vi "CAT071_main_org.vi"() -> ()   [LabVIEW 2015]
uses:
  class.dbc/controls/dbc-signal.ctl
  class.dbc/controls/dbc-frame.ctl
  class.dbc/controls/dbc-cluster.ctl
  class.can.table/CAN_table.ctl
  class.dbc/controls/signals.result.ctl
  class.dbc/controls/signal.result.ctl
  subs/frame.type.ctl
  class.bFrameIO/bFrameIO.lvclass/bFrameIO.ctl
  class.dbc/dbc.lvclass/dbc.ctl
  class.bFrameIO/controls/input-states.ctl
  class.dbc/Read-active-frame-tag.vi
  class.dbc/Read-active-item-symbol.vi
  class.dbc/Read-active-item-tag.vi
  class.bFrameIO/wrt-fi-state.vi
  class.dbc/Write-active-item-tag.vi
  class.dbc/Write-active-item-symbol.vi
  class.dbc/Write-active-item-indent-lvl.vi
  class.dbc/Write-active-frame-tag.vi
  class.bFrameIO/read-baud-rate.vi
  class.bFrameIO/wrt-device.vi
  class.bFrameIO/Read-frameQ.vi
  class.bFrameIO/wrt-baud-rate.vi
  class.dbc/dbc.lvclass
  class.bFrameIO/bFrameIO.lvclass
  LEDarray/LEDarray.lvclass
  class.can.table/bAPPdata.lvclass
panel:
  in  "Interface":refnum<k21>
  in  "dbc.alias":string="CAT071"
  out "Path":path caption="Open .dbc file"
  in  "CAT.071":enum32{"DBC", "table"}(tab)
  in  "attributes":T1(tab)
  out "CAN.table":T2
  out "dbc.cluster":T3={"Name"="", "Baud Rate"=125000, "Application Protocol"=enum."None", "Comment"=""}
  out "signal.results":T4 {"payload" format="%3d"}
  out "dbc.frame":T6={"Comment"="", "Extended Identifier?"=FALSE, "Transmit Time"=0.0, "Timing Type"=1, "Payload Length"=8, "Identifier"=1, "Frame name"="frame1"} {"Timing Type" items=["Cyclic Data", "Event Data", "Cyclic Remote", "Event Remote"]; "Identifier" format="%010x"}
  out "payload":bool[][](array[boolean])
  in  "send.frame":bool
  in  "frame.type":T7
  in  "send.signal":bool
  out "leds":picture
  out "output.signal":T8={"Comment"="", "Byte Order"=0, "Data Type"=1, "Number of Bits"=8, "Start Bit"=0, "Unit"="V", "Default Value"=0.0, "Minimum Value"=0.0, "Maximum Value"=256.0, "Scaling Offset"=0.0, "Scaling Factor"=1.0, "Signal name"="signal1"} {"Byte Order" items=["Little Endian", "Big Endian"]; "Data Type" items=["Signed", "Unsigned", "IEEE Float"]}
  out "signal.payload":u32
  in  "hslide":dbl(slide) min=0.0 max=250.0 scale=0.0..250.0
  out "output.signal 2":T8={"Comment"="", "Byte Order"=0, "Data Type"=1, "Number of Bits"=8, "Start Bit"=0, "Unit"="V", "Default Value"=0.0, "Minimum Value"=0.0, "Maximum Value"=256.0, "Scaling Offset"=0.0, "Scaling Factor"=1.0, "Signal name"="signal1"} {"Byte Order" items=["Little Endian", "Big Endian"]; "Data Type" items=["Signed", "Unsigned", "IEEE Float"]}
  out "signal.payload 2":u32 caption="signal.payload"
  out "payload 2":bool[][](array[boolean]) caption="payload"
  in  "database":string(tree)
  # "CAT 071 \nMarquardt Inc @2017\nK.R. Bergerstock"
  # "CLUSTER"
  # "FRAME"
  # "SIGNAL"
  # "SIGNAL"
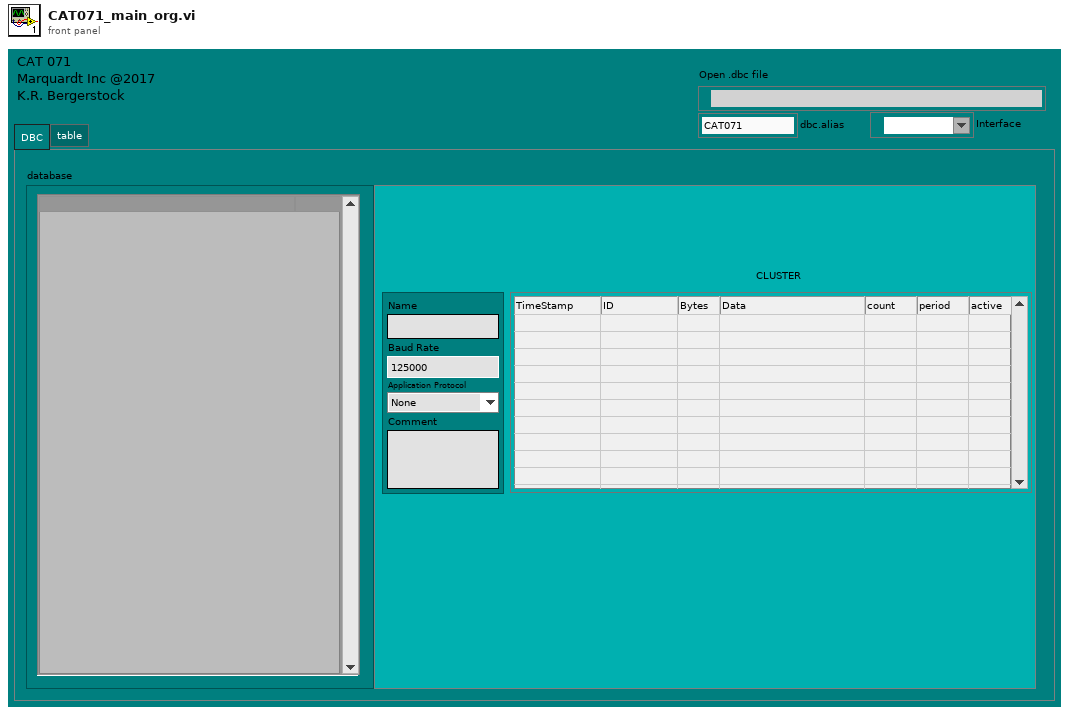
[diagram p1: front panel]
types:
  T1 = enum32{"cluster", "frame", "outp.signal", "inp.signal"}
  T2 = typedef "CAN_table.ctl" = string[][]
  T3 = typedef "dbc-cluster.ctl" = cluster{"Name":string, "Baud Rate":u32, "Application Protocol":enum16{"None", "J1939"}, "Comment":string}
  T4 = typedef "signals.result.ctl" = T5[]
  T5 = typedef "signal.result.ctl" = cluster{"Signal name":string, "payload":u8}
  T6 = typedef "dbc-frame.ctl" = cluster{"Comment":string, "Extended Identifier?":bool, "Transmit Time":dbl, "Timing Type":u32, "Payload Length":u32, "Identifier":u32, "Frame name":string}
  T7 = typedef "frame.type.ctl" = enum16{"FRAME NOT DEFINED", "DUT OUTPUT FRAME", "DUT INPUT FRAME"}
  T8 = typedef "dbc-signal.ctl" = cluster{"Comment":string, "Byte Order":u32, "Data Type":u32, "Number of Bits":u32, "Start Bit":u32, "Unit":string, "Default Value":dbl, "Minimum Value":dbl, "Maximum Value":dbl, "Scaling Offset":dbl, "Scaling Factor":dbl, "Signal name":string}
  T9 = typedef "bFrameIO.lvclass/input-states.ctl" = enum16{"idle", "start", "run", "stop", "exit"}
  T10 = typedef "frame-defination.ctl" = cluster{"CAN.frame":T6, "frame.type":T7}
  T11 = typedef "LVPoint32TypeDef.ctl" = cluster{"Horizontal":i32, "Vertical":i32}
  T12 = typedef "LVRectTypeDef.ctl" = cluster{"Left":i16, "Top":i16, "Right":i16, "Bottom":i16}
  T13 = typedef "XNET Frame CAN.ctl" = cluster{"timestamp":timestamp, "payload":u8[], "identifier":u32, "type":T14, "extended?":bool, "echo?":bool}
  T14 = typedef "XNET Frame Type CAN.ctl" = u8
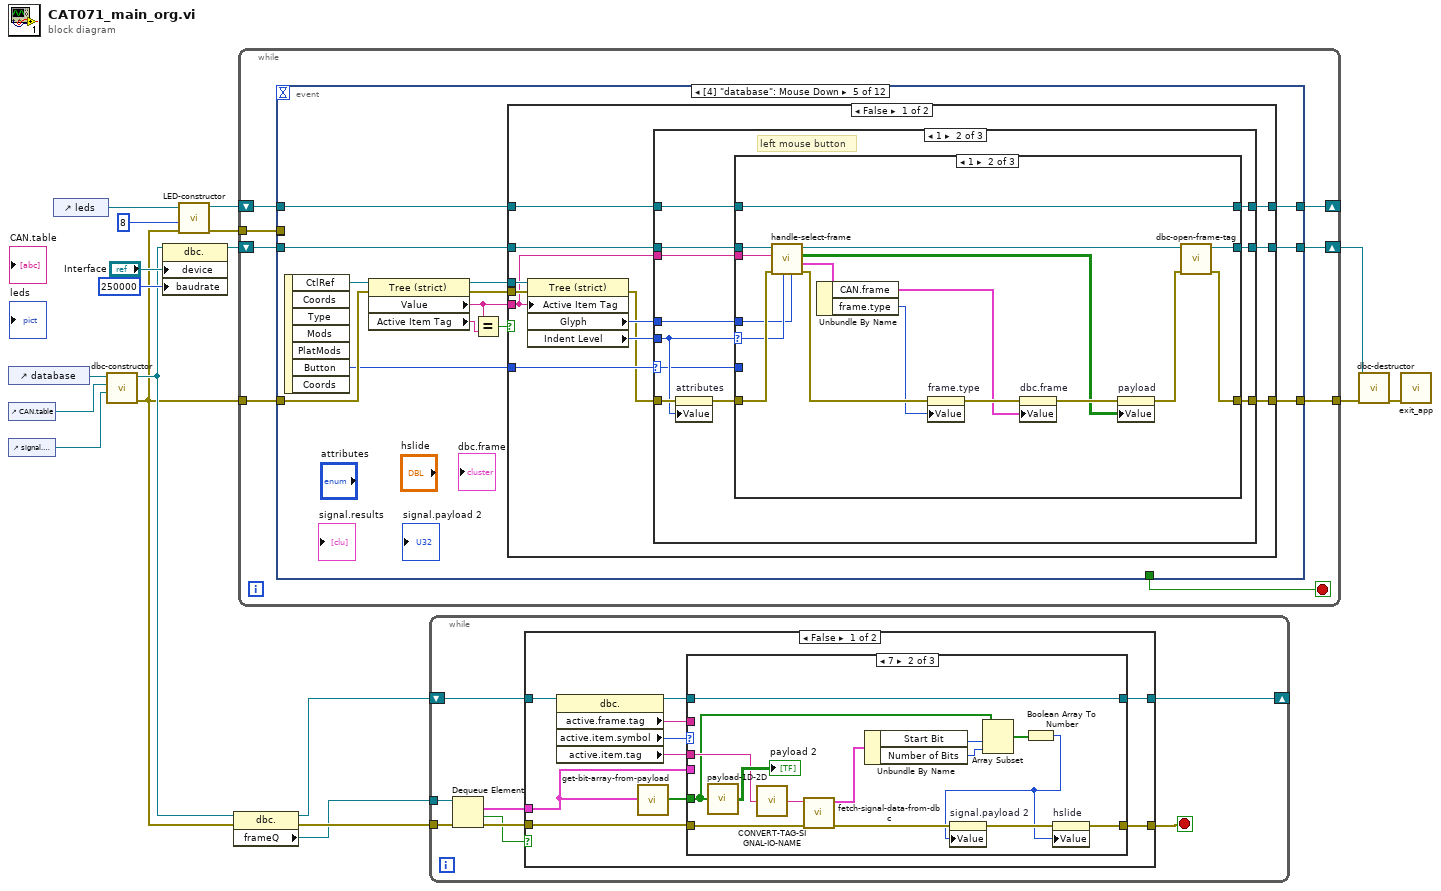
[diagram p0: block diagram]
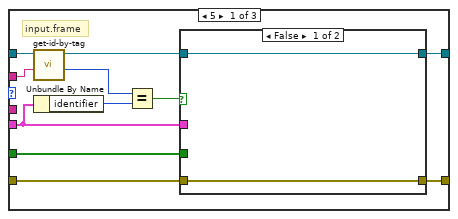
[diagram p2: hidden frame]
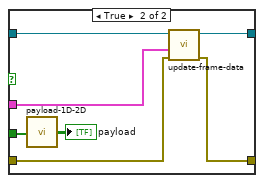
[diagram p3: hidden frame]
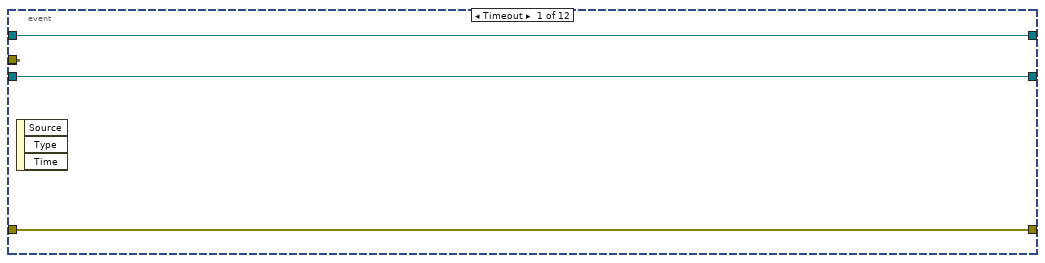
[diagram p6: hidden frame]
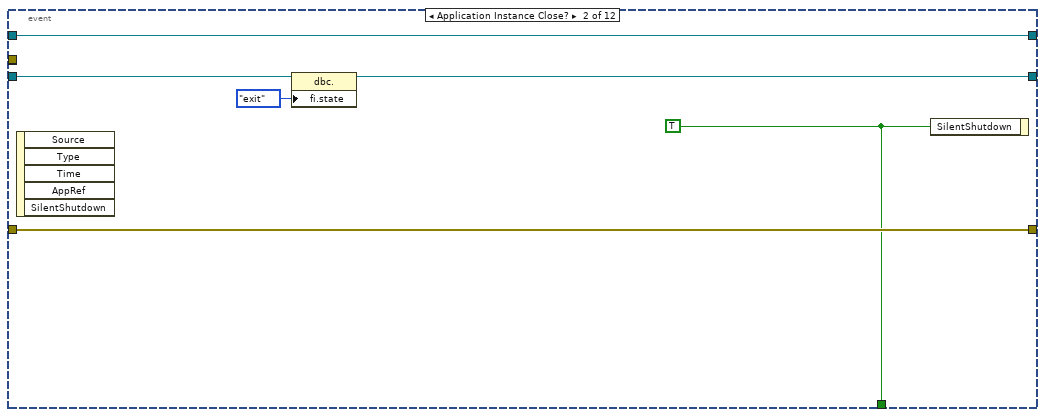
[diagram p7: hidden frame]
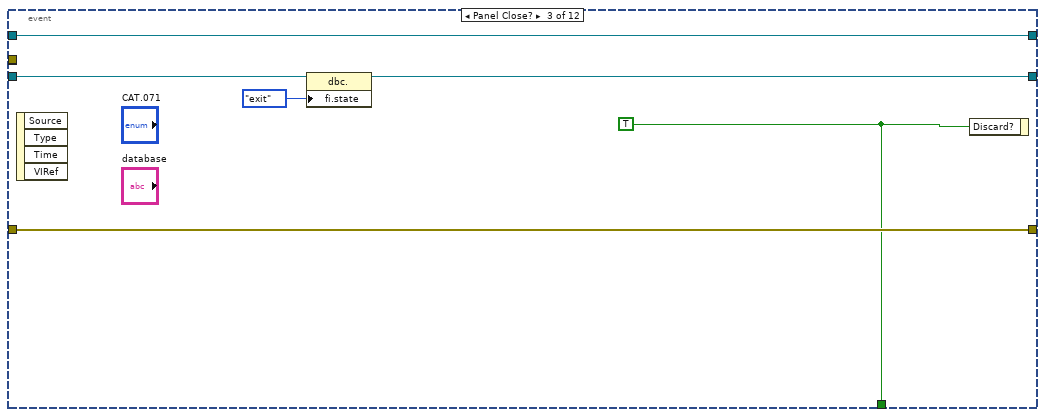
[diagram p8: hidden frame]
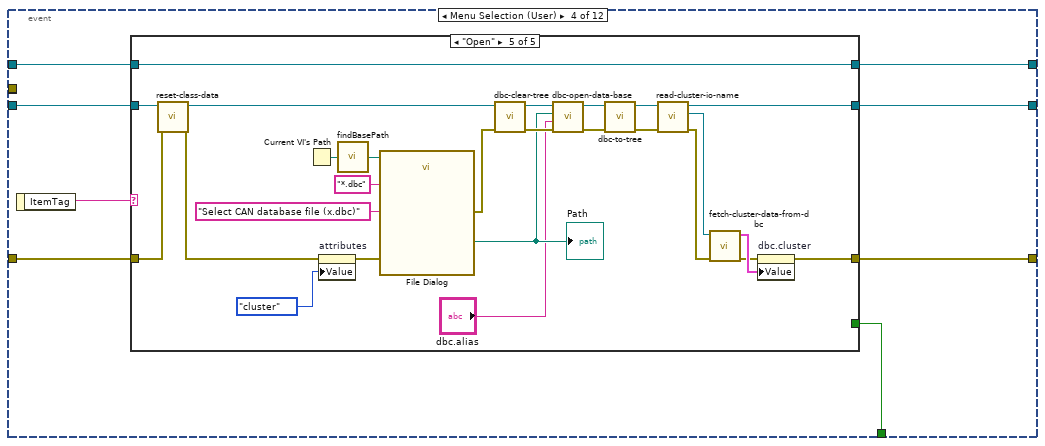
[diagram p9: hidden frame]
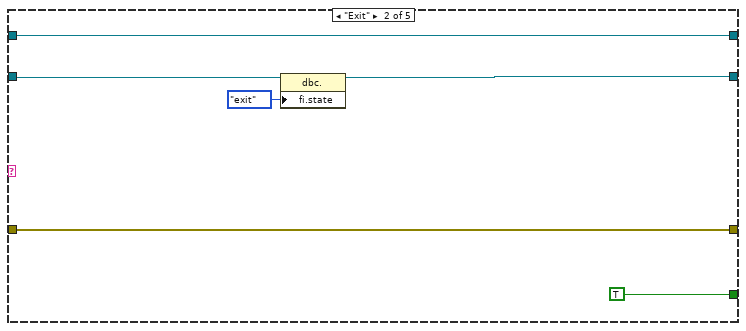
[diagram p11: hidden frame]
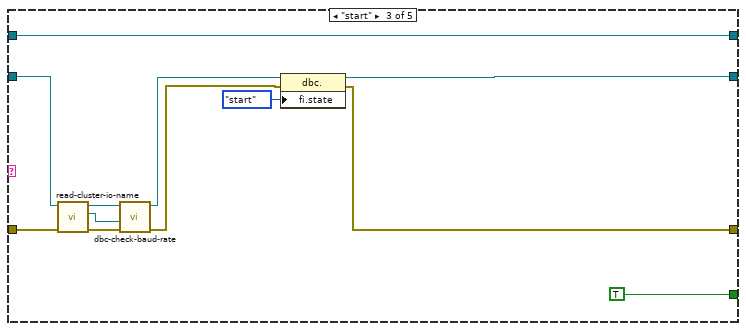
[diagram p12: hidden frame]
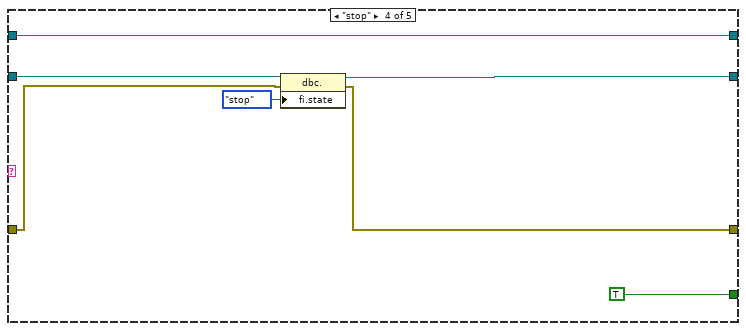
[diagram p13: hidden frame]
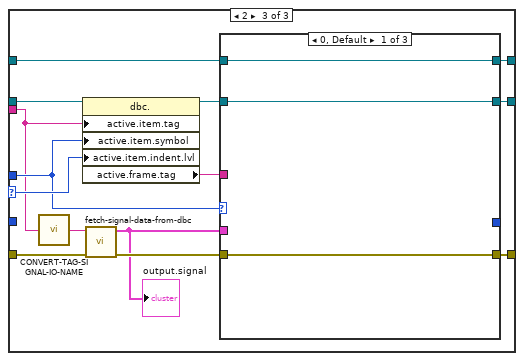
[diagram p16: hidden frame]
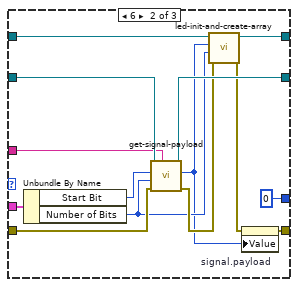
[diagram p17: hidden frame]
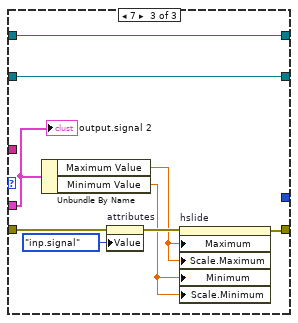
[diagram p18: hidden frame]
diagram:
  n1 = control-ref of="database"() -> (w17:refnum<vi>)
  n2 = control-ref of="CAN.table"() -> (w8:refnum<vi>)
  n3 = control-ref of="signal.results"() -> (w1:refnum<vi>)
  n4 = control-ref of="leds"() -> (w14:refnum<vi>)
  n5 = call "dbc-constructor.vi"("signal.results"=w1, "table.ref in"=w8, "tree.ref.in"=w17) -> ("error out"=w2:errorcluster, "dbc out"=w5:refnum<class "dbc.lvclass">)  [unwired: 7 in]
  n6 = property class="dbc."(reference=w5, "device"="Interface", "baudrate"=u32 250000) -> (reference out=w10:refnum<class "dbc.lvclass">)  [unwired: 1 in, 1 out]
  n7 = call "LED-constructor.vi"("error in (no error)"=w2, "radius"=8, "picture.ref"=w14) -> ("error out"=w11:errorcluster, "LEDarray out"=w12:refnum<class "LEDarray.lvclass">)  [unwired: 7 in]
  n8 = property class="dbc."(reference=w5, error in=w2) -> (reference out=w4:refnum<class "dbc.lvclass">, error out=w18:errorcluster, "frameQ"=w3:refnum<queue>)
  n9 = while {
    shift-right: [w26] -> w16
    shift-left: w10 -> [w25]
    tunnel: w2 -> [w24]
    tunnel: [w23] -> w9
    shift-right: [w20] -> _
    shift-left: w12 -> [w21]
    tunnel: w11 -> [w19]
    stop <- w22 stop-if-true
    n10 = event shown="[4] \"database\": Mouse Down" {
      selector: _ -> [_ _ _ _ _ _ _ _ _ _ _ _]
      dyn-events: _ -> [_ _ _ _ _ _ _ _ _ _ _ _]
      timeout: _ -> [_ _ _ _ _ _ _ _ _ _ _ _]
      tunnel: [w28 w33 w39 w46 w111 w212 w231 w279 w346 w364 w383 w388] -> w26
      tunnel: w25 -> [w28 w36 w42 w47 w112 w213 w230 w278 w346 w356 w375 w391]
      tunnel: w24 -> [w27 w35 w41 w48 w114 w215 w238 w286 w331 w371 w386 w390]
      tunnel: [w27 w35 w41 w49 w113 w214 w234 w282 w333 w361 w380 w390] -> w23
      tunnel: [_ w34 w40 w45 _ _ _ _ _ _ _ _] -> w22
      tunnel: w21 -> [w30 w31 w37 w44 w108 w216 w232 w280 w345 w370 w385 w389]
      tunnel: [w30 w31 w37 w43 w109 w216 w233 w281 w335 w370 w385 w389] -> w20
      tunnel: [w29 _ _ _ _ _ _ _ _ _ _ _] -> _
      tunnel: w19 -> [w29 _ _ _ _ _ _ _ _ _ _ _]
      event Timeout {
        n11 = event-data() -> ()  [unwired: 1 in, 3 out]
      }
      event Application Instance Close? {
        w34 = TRUE
        n12 = event-data() -> ()  [unwired: 1 in, 5 out]
        n13 = property class="dbc."(reference=w36, "fi.state"=input-states."exit") -> (reference out=w33:refnum<class "dbc.lvclass">)  [unwired: 1 in, 1 out]
        n14 = event-data("SilentShutdown"=w34) -> ()  [unwired: 1 in, 1 out]
      }
      event Panel Close? {
        w40 = TRUE
        n15 = event-data() -> ()  [unwired: 1 in, 4 out]
        n16 = property class="dbc."(reference=w42, "fi.state"=input-states."exit") -> (reference out=w39:refnum<class "dbc.lvclass">)  [unwired: 1 in, 1 out]
        n17 = event-data("Discard?"=w40) -> ()  [unwired: 1 in, 1 out]
      }
      event Menu Selection (User) {
        n18 = event-data() -> ("ItemTag"=w50:string)  [unwired: 1 in]
        n19 = case shown="\"Open\"" w50 {
          tunnel: [w53 w59 w60 w72 w93] -> w49
          tunnel: w48 -> [w53 w59 w64 w74 w81]
          tunnel: w47 -> [w52 w58 w63 w73 w82]
          tunnel: [w52 w56 w70 w77 w90] -> w46
          tunnel: [_ TRUE TRUE TRUE _] -> w45
          tunnel: w44 -> [w51 w54 w68 w75 w85]
          tunnel: [w51 w54 w68 w75 w85] -> w43
          frame Default {
          }
          frame "Exit" {
            n20 = property class="dbc."(reference=w58, "fi.state"=input-states."exit") -> (reference out=w56:refnum<class "dbc.lvclass">)  [unwired: 1 in, 1 out]
          }
          frame "start" {
            n21 = call "read-cluster-io-name.vi"("error in (no error)"=w64, "dbc in"=w63) -> ("error out"=w66:errorcluster, "XNET Cluster"=w65:refnum<k21>, "dbc out"=w67:refnum<class "dbc.lvclass">)  [unwired: 7 in]
            n22 = call "dbc-check-baud-rate.vi"("error in (no error)"=w66, "XNET Cluster 2"=w65, "dbc in"=w67) -> ("error out"=w61:errorcluster, "dbc out"=w62:refnum<class "dbc.lvclass">)  [unwired: 7 in]
            n23 = property class="dbc."(reference=w62, error in=w61, "fi.state"=input-states."start") -> (reference out=w70:refnum<class "dbc.lvclass">, error out=w60:errorcluster)
          }
          frame "stop" {
            n24 = property class="dbc."(reference=w73, error in=w74, "fi.state"=input-states."stop") -> (reference out=w77:refnum<class "dbc.lvclass">, error out=w72:errorcluster)
          }
          frame "Open" {
            n25 = call-dynamic "reset-class-data.vi"("error in (no error)"=w81, "CANtable in"=w82) -> ("error out"=w80:errorcluster, "CANtable out"=w84:refnum<class "dbc.lvclass">)  [unwired: 8 in]
            n26 = Current VI's Path() -> (path=w101:path)
            n27 = property on="attributes" class="TabCtl (strict)"(error in=w80, "Value"=T1."cluster" ("attributes")) -> (error out=w86:errorcluster)  [unwired: 1 in, 1 out]
            n28 = call "findBasePath.vi"("path.in"=w101) -> ("path.out"=w100:path)  [unwired: 4 in]
            n29 = call "File Dialog"("start path"=w100, "prompt"="Select CAN database file (x.dbc)", "error in"=w86, "pattern (all files)"="*.dbc") -> ("selected path"=w98:path, "error out"=w103:errorcluster)  [unwired: 8 in, 2 out]
            "Path" <- w98
            n30 = call "dbc-clear-tree.vi"("dbc in"=w84) -> ("dbc out"=w79:refnum<class "dbc.lvclass">)  [unwired: 9 in, 1 out]
            n31 = call "dbc-open-data-base.vi"("error in (no error)"=w103, "alias"="dbc.alias", "dbc.path"=w98, "dbc in"=w79) -> ("error out"=w94:errorcluster, "dbc out"=w99:refnum<class "dbc.lvclass">)  [unwired: 6 in]
            n32 = call "dbc-to-tree.vi"("error in (no error)"=w94, "dbc in"=w99) -> ("error out"=w88:errorcluster, "dbc out"=w95:refnum<class "dbc.lvclass">)  [unwired: 8 in]
            n33 = call "read-cluster-io-name.vi"("error in (no error)"=w88, "dbc in"=w95) -> ("error out"=w87:errorcluster, "XNET Cluster"=w89:refnum<k21>, "dbc out"=w90:refnum<class "dbc.lvclass">)  [unwired: 7 in]
            n34 = call "fetch-cluster-data-from-dbc.vi"("error in (no error)"=w87, "CLUSTER.TAG"=w89) -> ("error out"=w91:errorcluster, "CAN Cluster"=w92:T3)  [unwired: 8 in]
            n35 = property on="dbc.cluster" class="Clust (strict)"(error in=w91, "Value"=w92) -> (error out=w93:errorcluster)  [unwired: 1 in, 1 out]
          }
        }
      }
      event "database": Mouse Down {
        n36 = event-data() -> ("CtlRef"=w110:refnum<vi>, "Button"=w107:u16)  [unwired: 1 in, 5 out]
        n37 = property class="Tree (strict)"(reference=w110, error in=w114) -> (reference out=w116:refnum<vi>, error out=w115:errorcluster, "Value"=w106:string, "Active Item Tag"=w105:string)
        n38 = Equal?(x=w106, y=w105) -> (x = y?=w104:bool)
        n39 = case shown="False" w104 {
          tunnel: w116 -> [w127 _]
          tunnel: w115 -> [w126 w206]
          tunnel: [w125 w206] -> w113
          tunnel: w112 -> [w124 w207]
          tunnel: [w123 w207] -> w111
          tunnel: [w122 w208] -> w109
          tunnel: w108 -> [w121 w208]
          tunnel: w106 -> [w119 _]
          tunnel: w107 -> [w118 _]
          frame False {
            n40 = property class="Tree (strict)"(reference=w127, error in=w126, "Active Item Tag"=w119) -> (error out=w117:errorcluster, "Glyph"=w120:i32, "Indent Level"=w128:i32)  [unwired: 1 out]
            n41 = case shown="1" w118 {
              selector: w118 -> [_ w132 _]
              tunnel: w128 -> [_ w133 _]
              tunnel: w117 -> [w129 w135 w205]
              tunnel: [w129 w142 w205] -> w125
              tunnel: w124 -> [w131 w141 w204]
              tunnel: [w131 w140 w204] -> w123
              tunnel: [w130 w139 w203] -> w122
              tunnel: w121 -> [w130 w138 w203]
              tunnel: w120 -> [_ w137 _]
              tunnel: w119 -> [_ w136 _]
              frame 0, Default {
              }
              frame 1 {
                # "left mouse button"
                n42 = property on="attributes" class="TabCtl (strict)"(error in=w135, "Value"=w133) -> (error out=w134:errorcluster)  [unwired: 1 in, 1 out]
                n43 = case shown="1" w133 {
                  selector: w133 -> [_ w157 w167]
                  tunnel: w134 -> [w145 w159 w176]
                  tunnel: [w145 w146 w174] -> w142
                  tunnel: w141 -> [w144 w162 w172]
                  tunnel: [w144 w148 w173] -> w140
                  tunnel: w137 -> [_ w156 w166]
                  tunnel: [w143 w161 w171] -> w139
                  tunnel: w138 -> [w143 w161 w170]
                  tunnel: w136 -> [_ w158 w164]
                  tunnel: w132 -> [_ _ _]
                  frame Default {
                  }
                  frame 1 {
                    n44 = call "handle-select-frame.vi"("symbol"=w156, "Indent Level"=w157, "error in (no error)"=w159, "Tag"=w158, "dbc in"=w162) -> ("error out"=w155:errorcluster, "frame.def"=w151:T10, "payload"=w153:bool[][], "dbc out"=w160:refnum<class "dbc.lvclass">)  [unwired: 3 in]
                    n45 = Unbundle By Name(w151) -> ("CAN.frame"=w150:T6, "frame.type"=w149:T7)
                    n46 = property on="frame.type" class="Enum (strict)"(error in=w155, "Value"=w149) -> (error out=w152:errorcluster)  [unwired: 1 in, 1 out]
                    n47 = property on="dbc.frame" class="Clust (strict)"(error in=w152, "Value"=w150) -> (error out=w154:errorcluster)  [unwired: 1 in, 1 out]
                    n48 = property on="payload" class="Arr (strict)"(error in=w154, "Value"=w153) -> (error out=w147:errorcluster)  [unwired: 1 in, 1 out]
                    n49 = call "dbc-open-frame-tag.vi"("error in (no error)"=w147, "dbc in"=w160) -> ("error out"=w146:errorcluster, "dbc out"=w148:refnum<class "dbc.lvclass">)  [unwired: 8 in]
                  }
                  frame 2 {
                    n50 = call "CONVERT-TAG-SIGNAL-IO-NAME.vi"("tag"=w164) -> ("signal"=w163:string)  [unwired: 4 in]
                    n51 = property class="dbc."(reference=w172, "active.item.tag"=w164, "active.item.symbol"=w166, "active.item.indent.lvl"=w167) -> (reference out=w168:refnum<class "dbc.lvclass">, "active.frame.tag"=w165:string)  [unwired: 1 in, 1 out]
                    n52 = call "fetch-signal-data-from-dbc.vi"("error in (no error)"=w176, "signal.tag"=w163) -> ("error out"=w175:errorcluster, "can.signal"=w169:T8)  [unwired: 8 in]
                    "output.signal" <- w169
                    n53 = case shown="0, Default" w166 {
                      tunnel: w169 -> [_ w190 w197]
                      tunnel: w175 -> [w179 w188 w201]
                      tunnel: [w179 w182 w199] -> w174
                      tunnel: [w178 w189 w198] -> w173
                      tunnel: w168 -> [w178 w193 w198]
                      tunnel: [w177 w191 w202] -> w171
                      tunnel: w170 -> [w177 w192 w202]
                      tunnel: w165 -> [_ w186 _]
                      tunnel: [_ 0 _] -> _
                      frame 0, Default {
                      }
                      frame 6 {
                        n54 = Unbundle By Name(w190) -> ("Start Bit"=w185:u32, "Number of Bits"=w184:u32)
                        n55 = call "get-signal-payload.vi"("frame.tag"=w186, "error in (no error)"=w188, "bit.len"=w184, "start.pos"=w185, "CANtable in"=w193) -> ("error out"=w187:errorcluster, "payload"=w181:u32, "CANtable out"=w189:refnum<class "dbc.lvclass">)  [unwired: 4 in]
                        n56 = call "led-init-and-create-array.vi"("error in (no error)"=w187, "len.bits"=w184, "init.value"=w181, "LEDarray"=w192) -> ("error out"=w183:errorcluster, "LEDarray 2"=w191:refnum<class "LEDarray.lvclass">)  [unwired: 6 in]
                        n57 = property on="signal.payload" class="DigNum (strict)"(error in=w183, "Value"=w181) -> (error out=w182:errorcluster)  [unwired: 1 in, 1 out]
                      }
                      frame 7 {
                        n58 = Unbundle By Name(w197) -> ("Maximum Value"=w195:dbl, "Minimum Value"=w194:dbl)
                        n59 = property on="attributes" class="TabCtl (strict)"(error in=w201, "Value"=T1."inp.signal" ("attributes")) -> (error out=w200:errorcluster)  [unwired: 1 in, 1 out]
                        n60 = property on="hslide" class="Slide (strict)"(error in=w200, "Maximum"=w195, "Scale.Maximum"=w195, "Minimum"=w194, "Scale.Minimum"=w194) -> (error out=w199:errorcluster)  [unwired: 1 in, 1 out]
                        "output.signal 2" <- w197
                      }
                    }
                  }
                }
              }
              frame 2 {
                # "right mouse button"
              }
            }
          }
          frame True {
          }
        }
      }
      event Value Change {
        n61 = event-data() -> ("OldVal"=w211:T7, "NewVal"=w209:T7)  [unwired: 1 in, 4 out]
        n62 = Not Equal?(x=w211, y=w209) -> (x != y?=w210:bool)
        n63 = case shown="True" w210 {
          tunnel: w215 -> [w217 w226]
          tunnel: [w217 w225] -> w214
          tunnel: w213 -> [w218 w224]
          tunnel: [w218 w223] -> w212
          tunnel: w209 -> [_ w219]
          frame False {
          }
          frame True {
            n64 = property class="dbc."(reference=w224) -> (reference out=w222:refnum<class "dbc.lvclass">, "active.frame.tag"=w221:string)  [unwired: 1 in, 1 out]
            n65 = property on="dbc.frame" class="Clust (strict)"(error in=w226) -> (error out=w227:errorcluster, "Value"=w220:T6)  [unwired: 1 in, 1 out]
            n66 = call "dbc-mark-frame.vi"("CAN.frame"=w220, "tag"=w221, "error in (no error)"=w227, "action"=w219, "dbc in"=w222) -> ("error out"=w225:errorcluster, "dbc out"=w223:refnum<class "dbc.lvclass">)  [unwired: 5 in]
          }
        }
      }
      event "database": event #0x1e {
        n67 = event-data() -> ("CtlRef"=w239:refnum<vi>, "Tag"=w228:string)  [unwired: 1 in, 3 out]
        n68 = property class="Tree (strict)"(reference=w239, error in=w238, "Active Item Tag"=w228) -> (error out=w237:errorcluster, "Indent Level"=w236:i32, "Glyph"=w229:i32)  [unwired: 1 out]
        n69 = property on="attributes" class="TabCtl (strict)"(error in=w237, "Value"=w236) -> (error out=w235:errorcluster)  [unwired: 1 in, 1 out]
        n70 = case shown="1" w236 {
          selector: w236 -> [_ w251 w269]
          tunnel: w235 -> [w240 w255 w262]
          tunnel: [w240 w247 w272] -> w234
          tunnel: [w242 w258 w275] -> w233
          tunnel: w232 -> [w242 w258 w275]
          tunnel: [w241 w254 w274] -> w231
          tunnel: w230 -> [w241 w257 w260]
          tunnel: w229 -> [_ w250 w270]
          tunnel: w228 -> [_ w245 w271]
          frame Default {
          }
          frame 0 {
            w252 = ""
            n71 = call "dbc-close-frame-tag.vi"("error in (no error)"=w255, "dbc in"=w257) -> ("error out"=w253:errorcluster, "dbc out"=w256:refnum<class "dbc.lvclass">)  [unwired: 8 in]
            n72 = property class="dbc."(reference=w256, error in=w253, "active.frame.tag"=w252, "active.item.tag"=w252, "active.item.indent.lvl"=w251, "active.item.symbol"=w250) -> (reference out=w254:refnum<class "dbc.lvclass">, error out=w246:errorcluster, "baudrate"=w243:u32)
            n73 = call "fetch-cluster-data-from-dbc.vi"("error in (no error)"=w246, "CLUSTER.TAG"=w245) -> ("error out"=w248:errorcluster, "CAN Cluster"=w249:T3)  [unwired: 8 in]
            n74 = Bundle By Name(cluster=w249, "Baud Rate"=w243) -> (w244:T3)
            n75 = property on="dbc.cluster" class="Clust (strict)"(error in=w248, "Value"=w244) -> (error out=w247:errorcluster)  [unwired: 1 in, 1 out]
          }
          frame 1 {
            n76 = call "dbc-close-frame-tag.vi"("error in (no error)"=w262, "dbc in"=w260) -> ("error out"=w261:errorcluster, "dbc out"=w259:refnum<class "dbc.lvclass">)  [unwired: 8 in]
            n77 = call "handle-select-frame.vi"("symbol"=w270, "Indent Level"=w269, "error in (no error)"=w261, "Tag"=w271, "dbc in"=w259) -> ("error out"=w266:errorcluster, "frame.def"=w268:T10, "payload"=w273:bool[][], "dbc out"=w274:refnum<class "dbc.lvclass">)  [unwired: 3 in]
            n78 = Unbundle By Name(w268) -> ("CAN.frame"=w264:T6, "frame.type"=w263:T7)
            n79 = property on="dbc.frame" class="Clust (strict)"(error in=w266, "Value"=w264) -> (error out=w265:errorcluster)  [unwired: 1 in, 1 out]
            n80 = property on="frame.type" class="Enum (strict)"(error in=w265, "Value"=w263) -> (error out=w267:errorcluster)  [unwired: 1 in, 1 out]
            n81 = property on="payload" class="Arr (strict)"(error in=w267, "Value"=w273) -> (error out=w272:errorcluster)  [unwired: 1 in, 1 out]
          }
        }
      }
      event "database": Item Close {
        n82 = event-data() -> ("CtlRef"=w287:refnum<vi>, "Tag"=w276:string)  [unwired: 1 in, 3 out]
        n83 = property class="Tree (strict)"(reference=w287, error in=w286, "Active Item Tag"=w276) -> (error out=w285:errorcluster, "Indent Level"=w284:i32, "Glyph"=w277:i32)  [unwired: 1 out]
        n84 = property on="attributes" class="TabCtl (strict)"(error in=w285, "Value"=w284) -> (error out=w283:errorcluster)  [unwired: 1 in, 1 out]
        n85 = disable-structure shown="Enabled" {
          disable-tunnel: w284 -> [w295 _]
          disable-tunnel: w283 -> [w294 w327]
          disable-tunnel: [w293 w327] -> w282
          disable-tunnel: [w292 w328] -> w281
          disable-tunnel: w280 -> [w291 w328]
          disable-tunnel: [w290 w329] -> w279
          disable-tunnel: w278 -> [w289 w329]
          disable-tunnel: w277 -> [w288 _]
          frame Disabled {
            n86 = case shown="1" w295 {
              selector: w295 -> [_ w303 w315]
              tunnel: w294 -> [w296 w307 w316]
              tunnel: [w296 w301 w317] -> w293
              tunnel: [w298 w310 w326] -> w292
              tunnel: w291 -> [w298 w310 w326]
              tunnel: [w297 w306 w318] -> w290
              tunnel: w289 -> [w297 w309 w319]
              tunnel: w288 -> [_ w302 w314]
              frame Default {
              }
              frame 0 {
                (unwired) TRUE
                w304 = ""
                n87 = call "dbc-close-frame-tag.vi"("error in (no error)"=w307, "dbc in"=w309) -> ("error out"=w305:errorcluster, "dbc out"=w308:refnum<class "dbc.lvclass">)  [unwired: 8 in]
                n88 = property class="dbc."(reference=w308, error in=w305, "active.frame.tag"=w304, "active.item.tag"=w304, "active.item.indent.lvl"=w303, "active.item.symbol"=w302) -> (reference out=w306:refnum<class "dbc.lvclass">, error out=w300:errorcluster)
                n89 = property on="dbc.cluster" class="Clust (strict)"(error in=w300, "Value"=T3 {"Name"="", "Baud Rate"=125000, "Application Protocol"=enum."None", "Comment"=""} ("dbc.cluster")) -> (error out=w301:errorcluster)  [unwired: 1 in, 1 out]
              }
              frame 1 {
                w323 = ""
                n90 = call "dbc-close-frame-tag.vi"("error in (no error)"=w316, "dbc in"=w319) -> ("error out"=w324:errorcluster, "dbc out"=w322:refnum<class "dbc.lvclass">)  [unwired: 8 in]
                n91 = property on="dbc.frame" class="Clust (strict)"(error in=w324, "Value"=T6 {"Comment"="", "Extended Identifier?"=FALSE, "Transmit Time"=0.0, "Timing Type"=1, "Payload Length"=8, "Identifier"=1, "Frame name"="frame1"} ("dbc.frame")) -> (error out=w313:errorcluster)  [unwired: 1 in, 1 out]
                n92 = property class="dbc."(reference=w322, "active.item.tag"=w323, "active.frame.tag"=w323, "active.item.indent.lvl"=w315, "active.item.symbol"=w314) -> (reference out=w318:refnum<class "dbc.lvclass">, error out=w325:errorcluster)  [unwired: 1 in]
                n93 = property on="frame.type" class="Enum (strict)"(error in=w313, "Value"=frame.type."FRAME NOT DEFINED" ("frame.type")) -> (error out=w320:errorcluster)  [unwired: 1 in, 1 out]
                n94 = invoke on="payload" class="Arr (strict)" method="Reinit To Default"(error in=w320) -> (error out=w321:errorcluster)  [unwired: 2 in, 2 out]
                n95 = Merge Errors(w325, w321) -> (w317:errorcluster)
              }
            }
          }
          frame Enabled {
          }
        }
      }
      event "leds": Mouse Down {
        n96 = event-data() -> ("Coords"=w339:T11, "CtlRef"=w337:refnum<vi>)  [unwired: 1 in, 4 out]
        n97 = property class="Pict"(reference=w337, error in=w331) -> (error out=w330:errorcluster, "MasterRect"=w336:T12)  [unwired: 1 out]
        n98 = call "LED-get-location.vi"("error in (no error)"=w330, "MasterRect"=w336, "Coords"=w339, "LEDarray"=w345) -> ("error out"=w340:errorcluster, "y"=w341:i32, "x"=w342:i32, "LEDarray.out"=w344:refnum<class "LEDarray.lvclass">)  [unwired: 4 in]
        n99 = call "led-change-color.vi"("Color Box"=u32 3524608, "error in (no error)"=w340, "y"=w341, "x"=w342, "LEDarray"=w344) -> ("error out"=w334:errorcluster, "LEDarray 2"=w343:refnum<class "LEDarray.lvclass">)  [unwired: 5 in]
        n100 = call "LED-read-U32.vi"("error in (no error)"=w334, "LEDarray in"=w343) -> ("error out"=w333:errorcluster, "Numeric"=→"signal.payload":u32, "LEDarray out"=w335:refnum<class "LEDarray.lvclass">)  [unwired: 6 in, 1 out]
      }
      event "send.signal": Value Change {
        n101 = event-data() -> ()  [unwired: 1 in, 6 out]
        n102 = property on=".signal" class="Clust (strict)"(error in=w371) -> (error out=w349:errorcluster, "Value"=w369:T8)  [unwired: 1 in, 1 out]
        n103 = Unbundle By Name(w369) -> ("Number of Bits"=w353:u32, "Start Bit"=w354:u32)
        n104 = call "read-cluster-io-name.vi"("error in (no error)"=w349, "dbc in"=w356) -> ("error out"=w359:errorcluster, "XNET Cluster"=w358:refnum<k21>, "dbc out"=w360:refnum<class "dbc.lvclass">)  [unwired: 7 in]
        n105 = call "dbc-check-baud-rate.vi"("error in (no error)"=w359, "XNET Cluster 2"=w358, "dbc in"=w360) -> ("error out"=w348:errorcluster, "dbc out"=w357:refnum<class "dbc.lvclass">)  [unwired: 7 in]
        n106 = property on="signal.payload" class="DigNum (strict)"(error in=w348) -> (error out=w351:errorcluster, "Value"=w350:u32)  [unwired: 1 in, 1 out]
        n107 = Number To Boolean Array(number=w350) -> (Boolean array=w368:bool[])
        n108 = Reshape Array(w368, w353) -> (w352:bool[])
        n109 = property class="dbc."(reference=w357, error in=w351) -> (reference out=w355:refnum<class "dbc.lvclass">, error out=w372:errorcluster, "active.frame.tag"=w347:string)
        n110 = call "update-bit-payload-by-tag.vi"("CANtable in"=w355, "frame.tag"=w347, "Array"=w352, "start.pos"=w354, "error in (no error)"=w372) -> ("CANtable out"=w367:refnum<class "dbc.lvclass">, "error out"=w365:errorcluster)  [unwired: 9 in]
        n111 = call "get-new-can-frame-by-tag.vi"("error in (no error)"=w365, "tag"=w347, "CANtable in"=w367) -> ("error out"=w363:errorcluster, "CAN frame"=w362:T13, "CANtable out"=w366:refnum<class "dbc.lvclass">)  [unwired: 5 in, 1 out]
        n112 = call "output-frame.vi"("error in (no error)"=w363, "CAN frame"=w362, "fi in"=w366) -> ("error out"=w361:errorcluster, "fi out"=w364:refnum<class "dbc.lvclass">)  [unwired: 7 in]
      }
      event "send.frame": Value Change {
        n113 = event-data() -> ()  [unwired: 1 in, 6 out]
        n114 = call "read-cluster-io-name.vi"("dbc in"=w375) -> ("error out"=w378:errorcluster, "XNET Cluster"=w377:refnum<k21>, "dbc out"=w379:refnum<class "dbc.lvclass">)  [unwired: 8 in]
        n115 = call "dbc-check-baud-rate.vi"("error in (no error)"=w378, "XNET Cluster 2"=w377, "dbc in"=w379) -> ("dbc out"=w376:refnum<class "dbc.lvclass">)  [unwired: 7 in, 1 out]
        n116 = property class="dbc."(reference=w376) -> (reference out=w374:refnum<class "dbc.lvclass">, "active.frame.tag"=w373:string)  [unwired: 1 in, 1 out]
        n117 = call "get-new-can-frame-by-tag.vi"("error in (no error)"=w386, "tag"=w373, "CANtable in"=w374) -> ("error out"=w382:errorcluster, "CAN frame"=w381:T13, "CANtable out"=w384:refnum<class "dbc.lvclass">)  [unwired: 5 in, 1 out]
        n118 = call "output-frame.vi"("error in (no error)"=w382, "CAN frame"=w381, "fi in"=w384) -> ("error out"=w380:errorcluster, "fi out"=w383:refnum<class "dbc.lvclass">)  [unwired: 7 in]
      }
      event "Interface": Value Change {
        n119 = event-data() -> ("NewVal"=w387:refnum<k21>)  [unwired: 1 in, 5 out]
        n120 = property class="dbc."(reference=w391, "device"=w387) -> (reference out=w388:refnum<class "dbc.lvclass">)  [unwired: 1 in, 1 out]
      }
    }
  }
  n121 = while {
    tunnel: w3 -> [w398]
    tunnel: w18 -> [w393]
    shift-right: [w392] -> _
    shift-left: w4 -> [w399]
    stop <- w395 stop-if-true
    n122 = Dequeue Element(queue=w398, error in (no error)=w393) -> (element=w397:T13, timed out?=w394:bool, error out=w396:errorcluster)  [unwired: 1 in, 1 out]
    n123 = case shown="False" w394 {
      tunnel: [w409 w447] -> w395
      tunnel: w396 -> [w408 w447]
      tunnel: w397 -> [w402 _]
      tunnel: w399 -> [w407 w446]
      tunnel: [w406 w446] -> w392
      frame False {
        n124 = property class="dbc."(reference=w407) -> (reference out=w405:refnum<class "dbc.lvclass">, "active.frame.tag"=w403:string, "active.item.symbol"=w404:i32, "active.item.tag"=w400:string)  [unwired: 1 in, 1 out]
        n125 = call "get-bit-array-from-payload.vi"("CAN frame"=w402) -> ("Array"=w401:bool[])  [unwired: 4 in]
        n126 = case shown="7" w404 {
          tunnel: [w418 w440 w445] -> w409
          tunnel: w408 -> [w417 w437 w445]
          tunnel: w401 -> [w416 w434 _]
          tunnel: w402 -> [w411 _ _]
          tunnel: w405 -> [w420 w443 w444]
          tunnel: [w419 w443 w444] -> w406
          tunnel: w403 -> [w414 _ _]
          tunnel: w400 -> [_ w439 _]
          frame 5 {
            # "input.frame"
            n127 = call "get-id-by-tag.vi"("tag"=w414, "CANtable in"=w420) -> ("id"=w412:u32, "CANtable out"=w415:refnum<class "dbc.lvclass">)  [unwired: 7 in, 1 out]
            n128 = Unbundle By Name(w411) -> ("identifier"=w410:u32)
            n129 = Equal?(x=w412, y=w410) -> (x = y?=w413:bool)
            n130 = case shown="False" w413 {
              tunnel: [w421 w428] -> w419
              tunnel: [w422 w427] -> w418
              tunnel: w417 -> [w422 w426]
              tunnel: w416 -> [_ w425]
              tunnel: w411 -> [_ w424]
              tunnel: w415 -> [w421 w423]
              frame False {
              }
              frame True {
                n131 = call "payload-1D-2D.vi"("Array"=w425) -> ("Array 2"=→"payload":bool[][])  [unwired: 4 in]
                n132 = call "update-frame-data.vi"("error in (no error)"=w426, "id"=w424, "dbc in"=w423) -> ("error out"=w427:errorcluster, "dbc out"=w428:refnum<class "dbc.lvclass">)  [unwired: 6 in, 1 out]
              }
            }
          }
          frame 7 {
            n133 = call "payload-1D-2D.vi"("Array"=w434) -> ("Array 2"=→"payload 2":bool[][])  [unwired: 4 in]
            n134 = call "CONVERT-TAG-SIGNAL-IO-NAME.vi"("tag"=w439) -> ("signal"=w438:string)  [unwired: 4 in]
            n135 = call "fetch-signal-data-from-dbc.vi"("error in (no error)"=w437, "signal.tag"=w438) -> ("error out"=w436:errorcluster, "can.signal"=w435:T8)  [unwired: 8 in]
            n136 = Unbundle By Name(w435) -> ("Start Bit"=w433:u32, "Number of Bits"=w432:u32)
            n137 = Array Subset(array=w434, index=w433, length=w432) -> (w431:bool[])
            n138 = Boolean Array To Number(Boolean array=w431) -> (number=w430:u32)
            n139 = property on="signal.payload 2" class="DigNum (strict)"(error in=w436, "Value"=w430) -> (error out=w441:errorcluster)  [unwired: 1 in, 1 out]
            n140 = property on="hslide" class="Slide (strict)"(error in=w441, "Value"=w430) -> (error out=w440:errorcluster)  [unwired: 1 in, 1 out]
          }
          frame Default {
          }
        }
      }
      frame True {
      }
    }
  }
  n141 = call "dbc-destructor.vi"("error in (no error)"=w9, "dbc in"=w16) -> ("error out"=w15:errorcluster)  [unwired: 9 in]
  n142 = call "exit_app.vi"("error in (no error)"=w15) -> ()  [unwired: 11 in]
